vi "Main.vi"() -> ()   [LabVIEW 2018]
uses:
  <vilib>/Platform/TimedLoop/XDataNode/timing_clust.ctl
  <vilib>/Platform/TimedLoop/XDataNode/nitl_modes.ctl
  <vilib>/Platform/TimedLoop/XDataNode/wakeup.ctl
  <vilib>/myRIO/Instrument Drivers/Onboard IO/I2C/vis/Configure.vi
  <vilib>/myRIO/Instrument Drivers/Onboard IO/I2C/vis/Write.vi
  <vilib>/myRIO/Instrument Drivers/Onboard IO/DIO/vis/Read.vi
  <vilib>/myRIO/Instrument Drivers/Onboard IO/I2C/vis/Write Read.vi
  <vilib>/myRIO/Common/Instrument Driver Framework/myRIO v1.0/UART/vis/myRIO v1.0 Close UART.vi
  <vilib>/myRIO/Instrument Drivers/Onboard IO/I2C/vis/Smart Open.vi
  <vilib>/Utility/error.llb/Error Cluster From Error Code.vi
  <vilib>/myRIO/Common/Instrument Driver Framework/myRIO v1.0/I2C/vis/myRIO v1.0 Configure I2C.vi
  <vilib>/myRIO/Common/Instrument Driver Framework/myRIO v1.0/I2C/vis/myRIO v1.0 Write I2C.vi
  <vilib>/myRIO/Instrument Drivers/Onboard IO/DIO/vis/Smart Open.vi
  <vilib>/myRIO/Common/Instrument Driver Framework/myRIO v1.0/DIO/vis/myRIO v1.0 Read DIO.vi
  <vilib>/myRIO/Common/Instrument Driver Framework/myRIO v1.0/I2C/vis/myRIO v1.0 Read I2C.vi
  <vilib>/myRIO/Common/Instrument Driver Framework/Utilities/vis/FPGA Ref Manager.vi
  <vilib>/myRIO/Common/Instrument Driver Framework/myRIO v1.0/myRIO v1.0 Reset FPGA.vi
  <vilib>/myRIO/Common/Instrument Driver Framework/myRIO v1.0/IRQ/vis/myRIO v1.0 IRQ Info FGV.vi
  <vilib>/myRIO/Common/Instrument Driver Framework/myRIO v1.0/IRQ/vis/myRIO v1.0 Timer IRQ Info FGV.vi
  <vilib>/myRIO/Common/Instrument Driver Framework/myRIO v1.0/IRQ/vis/myRIO v1.0 ISR Agent.vi
  <vilib>/Platform/TimedLoop/XDataNode/XDataNode.xnode
  <vilib>/myRIO/Instrument Drivers/Utilities/Utilities.lvlib
  <vilib>/Platform/TimedLoop/XDataNode/XDNodeRunTimeDep.lvlib
panel:
  out "Magnetic field [LSb]":cluster{i16, i16, i16}(graph) caption="Waveform Chart"
  out "Z":i16
  out "Y":i16
  out "X":i16
  out "DATA":u8[](array[numeric]) format="%02x"
  in  "[ESC]":bool
  # "Compass demo"
  # "DATA_X_H"
  # "DATA_X_L"
  # "DATA_Z_H"
  # "DATA_Z_L"
  # "DATA_Y_H"
  # "DATA_Y_L"
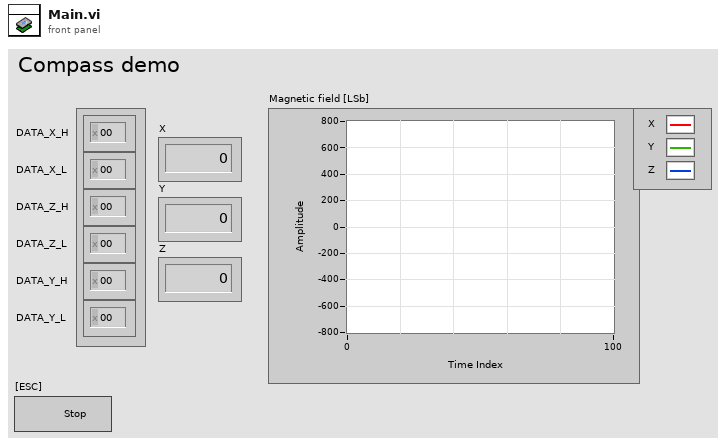
[diagram p1: front panel]
types:
  T1 = typedef "XDNodeRunTimeDep.lvlib/timing_clust.ctl" = cluster{"Expected End [f-1]":u64, "Actual End [f-1]":u64, "Finished Late? [f-1]":bool, "Expected End [i-1]":u64, "Actual End [i-1]":u64, "Finished Late? [i-1]":bool, "Expected Start [i]":u64, "Actual Start [i]":u64, "Expected Start [f]":u64, "Actual Start [f]":u64, "Source Name":string, "Structure Name":string, "Period":i64, "Deadline":i64, "Offset":i64, "Start":i64, "Priority":i32, "Timeout":i32, "Mode":T2, "Wakeup Reason":T3, "Error":errorcluster, "Source Type":string, "Secondary Source Type":string, "Global End Time":u64, "Global Start Time":u64, "Frame Duration":u64, "Iteration Duration":u64, "Assigned CPU":i32, "I/O Scan Engine Mode":u32}
  T2 = typedef "XDNodeRunTimeDep.lvlib/nitl_modes.ctl" = enum32{"No Change", "Process missed periods, maintain original phase", "Discard missed periods, maintain original phase", "Process missed periods, ignore original phase", "Discard missed periods, ignore original phase"}
  T3 = typedef "XDNodeRunTimeDep.lvlib/wakeup.ctl" = enum32{"Normal", "Aborted", "Asynchronous wakeup", "Timing source error", "Timed loop error", "Timeout"}
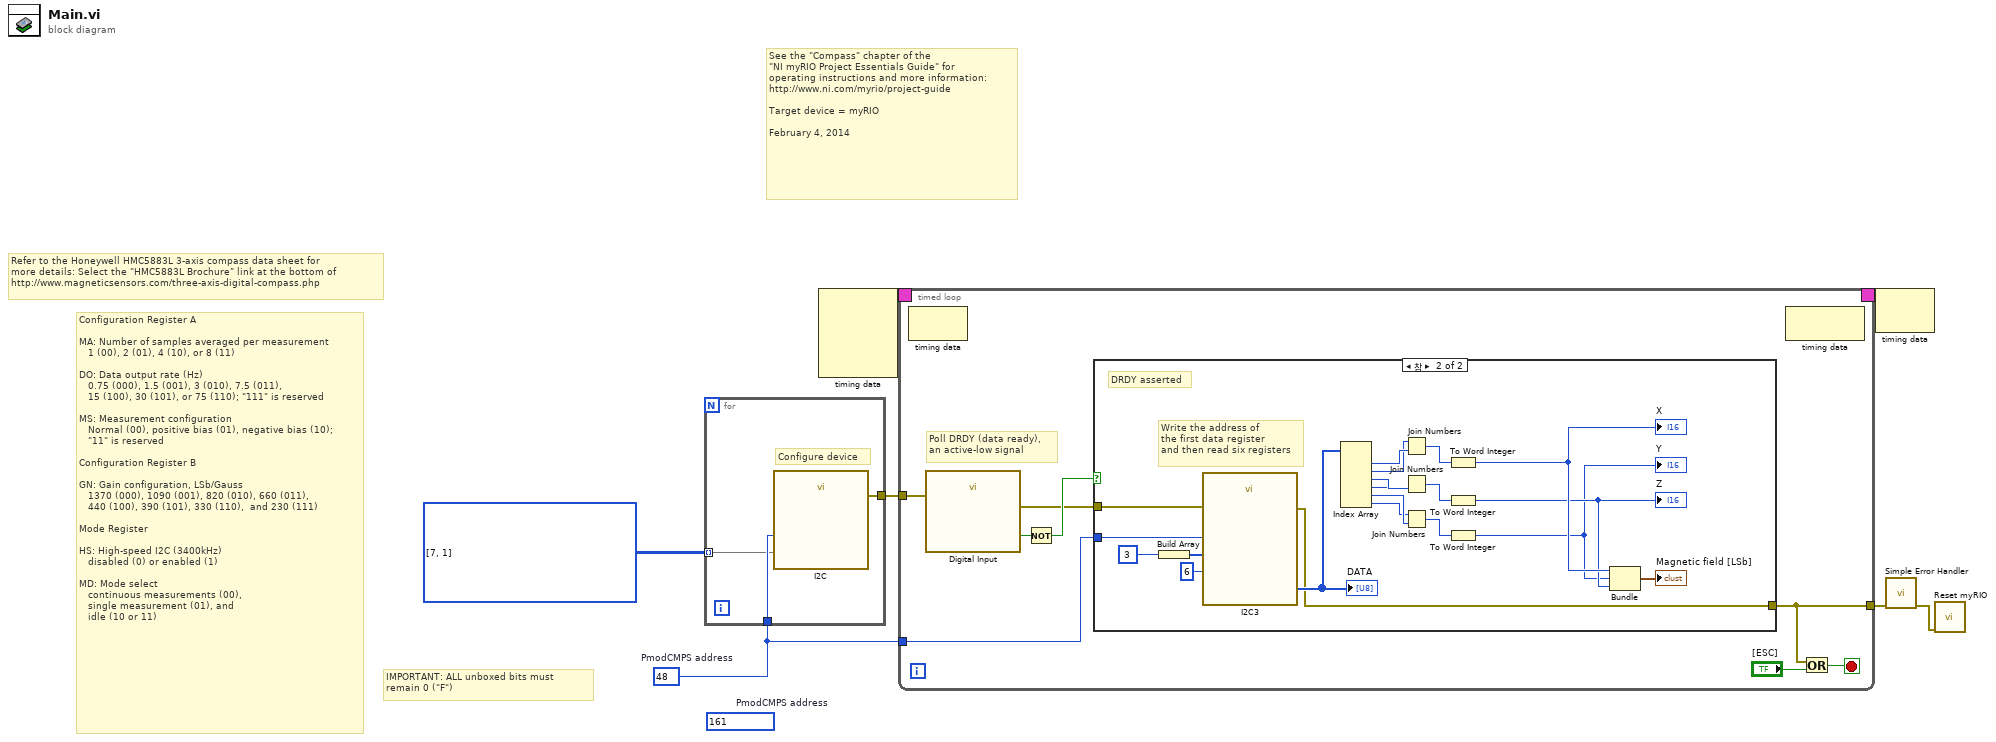
[diagram p0: block diagram]
diagram:
  (unwired) u8 161  # PmodCMPS address
  w4 = u8 48  # PmodCMPS address
  # "See the \"Compass\" chapter of the\n\"NI myRIO Project Essentials Guide\" for\noperating instructions and more information: \nhttp://www.ni.com/myrio/project-guide\n\nTarget device = myRIO\n\nFebruary 4, 2014"
  # "Refer to the Honeywell HMC5883L 3-axis compass data sheet for \nmore details: Select the \"HMC5883L Brochure\" link at the bottom of\nhttp://www.magneticsensors.com/three-axis-digital-compass.php"
  # "Configuration Register A\n\nMA: Number of samples averaged per measurement\n   1 (00), 2 (01), 4 (10), or 8 (11)\n\nDO: Data output rate (Hz)\n   0.75 (000), 1.5 (001), 3 (010), 7.5 (011),\n   15 (100), 30 (101), or 75 (110); \"111\" is reserved\n\nMS: Measurement configuration\n   Normal (00), positive bias (01), negative bias (10);\n   \"11\" is reserved\n\nConfiguration Register B\n\nGN: Gain configuration, LSb/Gauss\n   1370 (000), 1090 (001), 820 (010), 660 (011),\n   440 (100), 390 (101), 330 (110),  and 230 (111)\n\nMode Register\n\nHS: High-speed I2C (3400kHz)\n   disabled (0) or enabled (1)\n\nMD: Mode select\n   continuous measurements (00),\n   single measurement (01), and\n   idle (10 or 11)"
  # "IMPORTANT: ALL unboxed bits must\nremain 0 (\"F\")"
  n1 = for {
    tunnel: [w10] -> w5
    tunnel: w4 -> [w9]
    tunnel: u8[][] [[7, 1]] ("Bytes to Write") -> [w8] mode=indexing
    # "Configure device"
    n2 = call "I2C"("Slave Address (7-bit)"=w9, "Bytes to Write"=w8) -> ("error out"=w10:errorcluster)  [unwired: 25 in]
  }
  n3 = node-c288() -> (w3:T1)  [unwired: 4 in]
  n4 = timed-loop {
    tunnel: [w11] -> w6
    tunnel: w5 -> [w15]
    tunnel: w4 -> [w16]
    timing: w3 -> [_]
    timing-out: [_] -> w2
    stop <- w18 stop-if-true
    # "Poll DRDY (data ready),\nan active-low signal"
    n5 = node-c288() -> ()  [unwired: 1 in, 1 out]
    n6 = call "Digital Input"("error in (no error)"=w15) -> ("A/DIO0 (Pin 11)"=w14:bool, "error out"=w12:errorcluster)  [unwired: 25 in]
    n7 = Not(x=w14) -> (.not. x?=w13:bool)
    n8 = case shown="참" w13 {
      tunnel: w16 -> [_ w41]
      tunnel: w12 -> [w21 w30]
      tunnel: [w21 w26] -> w11
      frame False {
        # "DRDY deasserted"
      }
      frame True {
        # "DRDY asserted"
        # "Write the address of\nthe first data register\nand then read six registers"
        n9 = Build Array(u8 3) -> (w27:u8[])
        n10 = call "I2C3"("Slave Address (7-bit)"=w41, "Bytes to Write"=w27, "Byte Count"=u32 6, "error in (no error)"=w30) -> ("Bytes Read"=w31:u8[], "error out"=w26:errorcluster)  [unwired: 22 in]
        "DATA" <- w31
        n11 = Index Array "Index Array"(array=w31) -> (element #1=w40:u8, element #2=w39:u8, element #3=w37:u8, element #4=w36:u8, element #5=w35:u8, element #6=w34:u8)  [unwired: 6 in]
        n12 = Join Numbers(hi=w39, lo=w40) -> ((hi.lo)=w38:u16)
        n13 = Join Numbers(hi=w36, lo=w37) -> ((hi.lo)=w33:u16)
        n14 = Join Numbers(hi=w34, lo=w35) -> ((hi.lo)=w32:u16)
        n15 = To Word Integer(number=w38) -> (16bit integer=w24:i16)
        "X" <- w24
        n16 = To Word Integer(number=w33) -> (16bit integer=w23:i16)
        "Z" <- w23
        n17 = To Word Integer(number=w32) -> (16bit integer=w22:i16)
        "Y" <- w22
        n18 = Bundle(w24, w22, w23) -> (→"Magnetic field [LSb]":cluster{i16, i16, i16})  [unwired: 1 in]
      }
    }
    n19 = node-c288() -> ()  [unwired: 1 in, 1 out]
    n20 = Or(x=w11, y="[ESC]") -> (x .or. y?=w18:bool)
  }
  n21 = node-c288(w2) -> ()  [unwired: 1 out]
  n22 = call <vilib>:"Simple Error Handler.vi"("error in (no error)"=w6) -> ("error out"=w7:errorcluster)  [unwired: 4 in, 4 out]
  n23 = call <vilib>:"Reset myRIO.vi"("error in (no error)"=w7) -> ()  [unwired: 10 in, 1 out]
